vi "Create Exp Seg.vi"(6 "Number of Points":i32=100, 7 "Y 2":dbl(slide) scale=0.1..10.0, 8 "X 2":dbl(slide) scale=0.0..10.0, 9 "Y 1":dbl(slide) scale=0.1..10.0, 10 "X 1":dbl(slide) scale=0.0..10.0) -> (3 "Line Segment":cluster{dbl[], dbl[]}(graph))   [LabVIEW 2012]
uses:
  <vilib>/Analysis/NI_AALPro.lvlib
panel:
  in  "Sharpness":dbl(knob)=2.718281828459045 scale=0.5..1000.0
  out "Best Exponential Fit":dbl[](array[numeric])
  out "damping":dbl
  out "offset":dbl
  out "amplitude":dbl
  out "error out":errorcluster
  out "Plot With Point Markers":cluster{dbl[], dbl[]}[](graph)
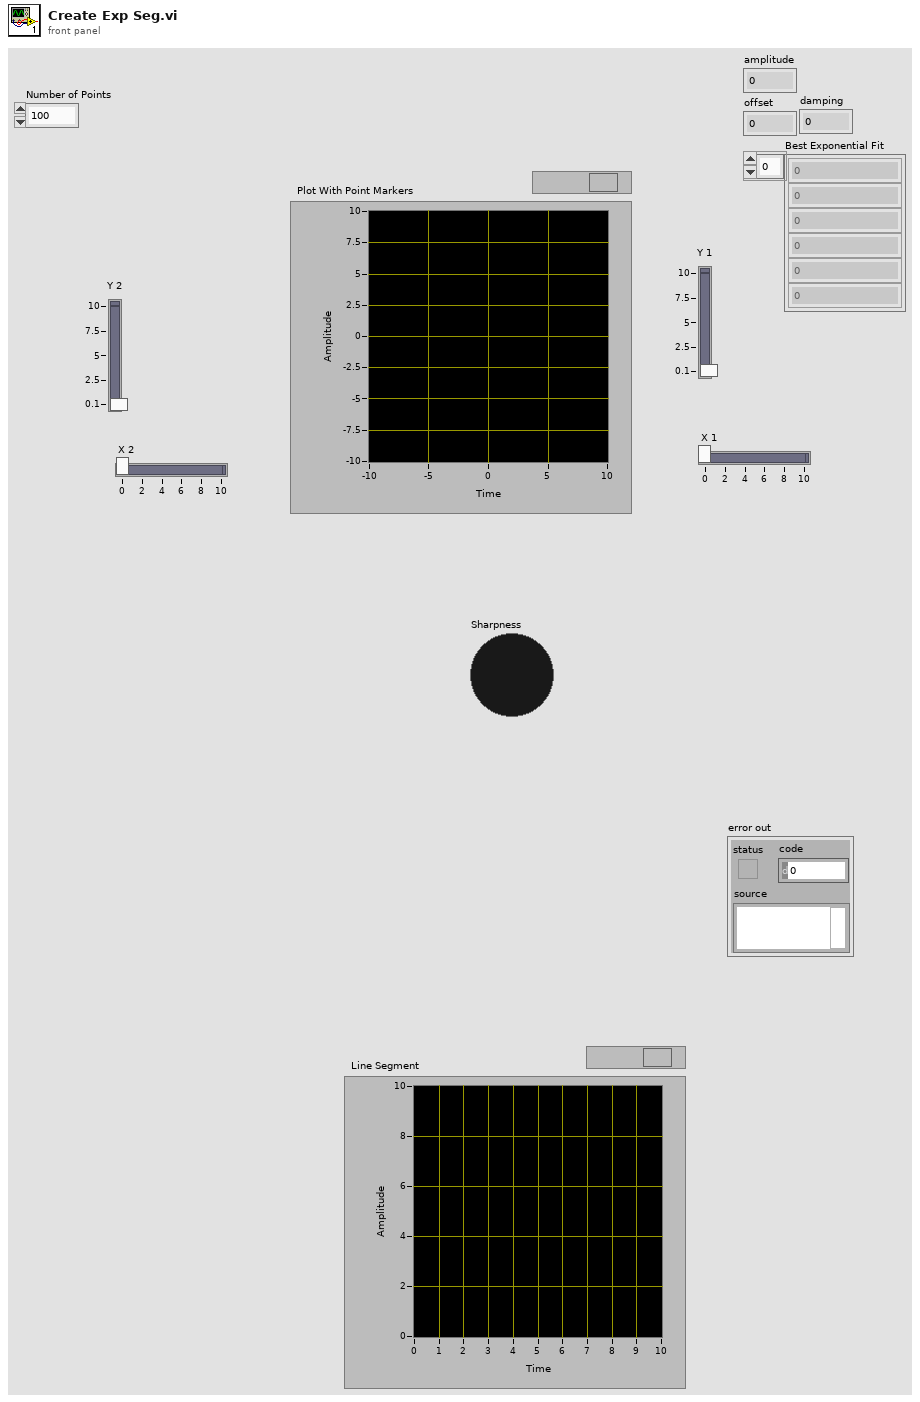
[diagram p1: front panel]
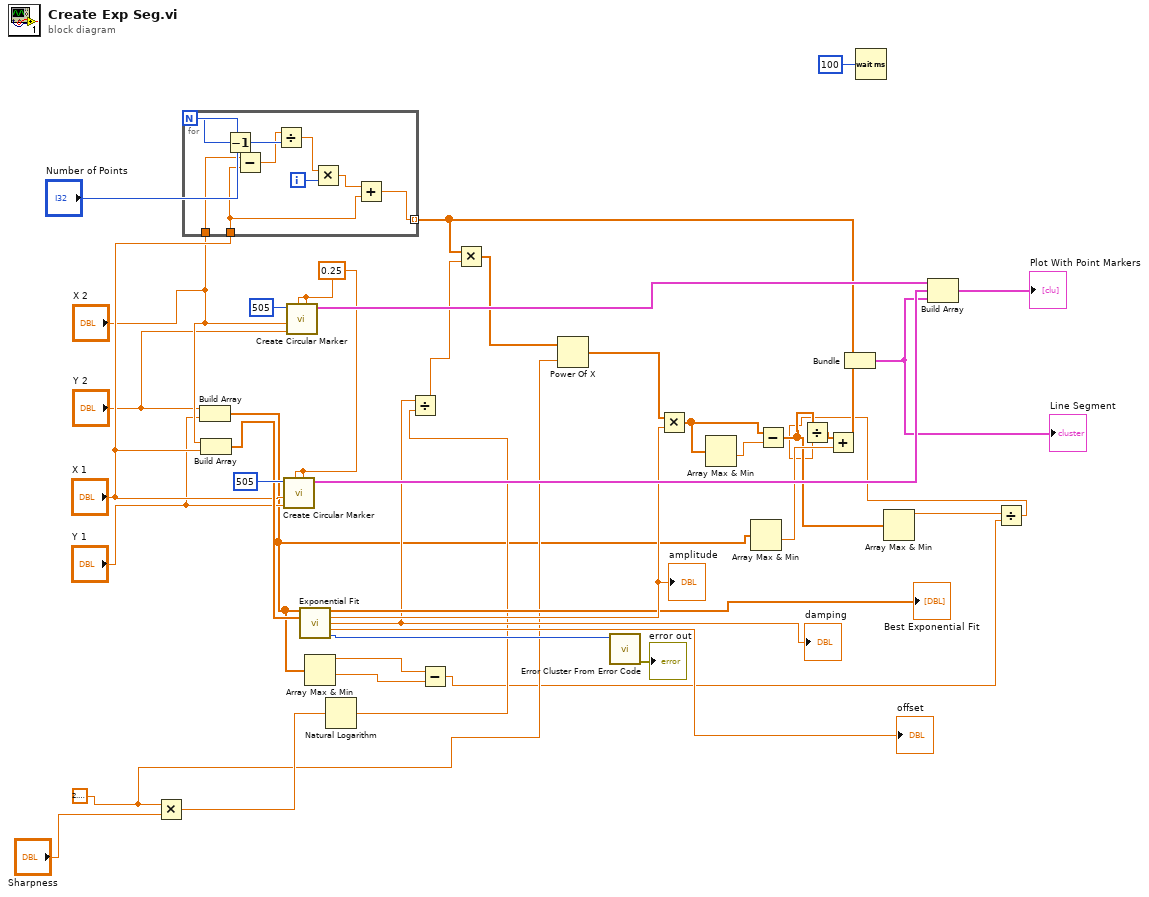
[diagram p0: block diagram]
diagram:
  w11 = 2.718281828459045
  w33 = 0.25 ("X Radius")
  n1 = Multiply(x=w11, y="Sharpness") -> (x*y=w12:dbl)
  n2 = for {
    N: "Number of Points" -> [w49]
    tunnel: [w44] -> w9 mode=indexing
    tunnel: "X 2" -> [w45]
    tunnel: "X 1" -> [w43]
    i -> [w47]
    n3 = Decrement(x=w49) -> (x-1=w42:i32)
    n4 = Subtract(x=w45, y=w43) -> (x-y=w41:dbl)
    n5 = Divide(x=w41, y=w42) -> (x/y=w48:dbl)
    n6 = Multiply(x=w48, y=w47) -> (x*y=w46:dbl)
    n7 = Add(x=w46, y=w43) -> (x+y=w44:dbl)
  }
  n8 = Build Array("Y 2", "Y 1") -> (w7:dbl[])
  n9 = Build Array("X 2", "X 1") -> (w34:dbl[])
  n10 = call "Create Circular Marker.vi"("Y Radius"=w33, "X Radius"=w33, "Y Center"="Y 1", "X Center"="X 1", "Number of Points"=505) -> ("XY Graph"=w39:cluster{dbl[], dbl[]})  [unwired: 6 in]
  n11 = call "Create Circular Marker.vi"("Y Radius"=w33, "X Radius"=w33, "Y Center"="Y 2", "X Center"="X 2", "Number of Points"=505) -> ("XY Graph"=w37:cluster{dbl[], dbl[]})  [unwired: 6 in]
  n12 = call <vilib>:"Exponential Fit.vi"("Y"=w7, "X"=w34) -> ("Best Exponential Fit"=→"Best Exponential Fit":dbl[], "amplitude"=w27:dbl, "damping"=w15:dbl, "offset"=→"offset":dbl, "error"=w32:i32)  [unwired: 8 in, 1 out]
  "amplitude" <- w27
  "damping" <- w15
  n13 = Array Max & Min(array=w7) -> (max value=w6:dbl, min value=w8:dbl)  [unwired: 2 out]
  n14 = Natural Logarithm(1:w12) -> (0:w14:dbl)
  n15 = Divide(x=w15, y=w14) -> (x/y=w16:dbl)
  n16 = Subtract(x=w6, y=w8) -> (x-y=w4:dbl)
  n17 = Multiply(x=w9, y=w16) -> (x*y=w17:dbl[])
  n18 = Power Of X(1:w11, 2:w17) -> (0:w18:dbl[])
  n19 = call <vilib>:"Error Cluster From Error Code.vi"("error code (0)"=w32) -> ("error out"=→"error out":errorcluster)  [unwired: 8 in]
  n20 = Multiply(x=w18, y=w27) -> (x*y=w25:dbl[])
  n21 = Array Max & Min(array=w25) -> (min value=w26:dbl)  [unwired: 3 out]
  n22 = Array Max & Min(array=w7) -> (min value=w21:dbl)  [unwired: 3 out]
  n23 = Subtract(x=w25, y=w26) -> (x-y=w2:dbl[])
  n24 = Wait (ms)(milliseconds to wait=u32 100) -> ()  [unwired: 1 out]
  n25 = Array Max & Min(array=w2) -> (max value=w5:dbl)  [unwired: 3 out]
  n26 = Divide(x=w5, y=w4) -> (x/y=w1:dbl)
  n27 = Divide(x=w2, y=w1) -> (x/y=w3:dbl[])
  n28 = Add(x=w3, y=w21) -> (x+y=w23:dbl[])
  n29 = Bundle(w9, w23) -> (w24:cluster{dbl[], dbl[]})  [unwired: 1 in]
  "Line Segment" <- w24
  n30 = Build Array(w37, w39, w24) -> (→"Plot With Point Markers":cluster{dbl[], dbl[]}[])
